vi "DC Supply Control.vi"(8 "error in":errorcluster, 10 "VISA res in":refnum<visa-resource-name>, 11 "HTS Results in":refnum<class "HTS Results.lvclass">) -> (0 "error out":errorcluster, 1 "Supp I":dbl, 2 "VISA res out":refnum<visa-resource-name>, 3 "HTS Results out":refnum<class "HTS Results.lvclass">)   [LabVIEW 2019, in "Results.lvlib" / "HTS Results.lvclass"]
uses:
  HTS Results.lvclass
  HTS Results.lvclass/HTS Results.ctl
  <instrlib>/Agilent 66XX Series/Agilent 66XX Series.lvlib
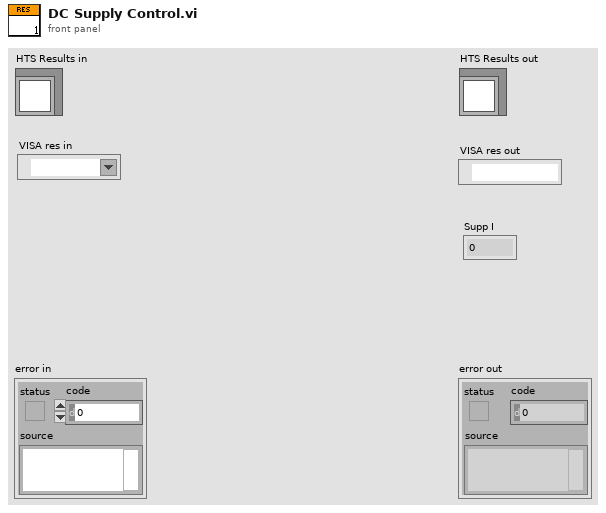
[diagram p1: front panel]
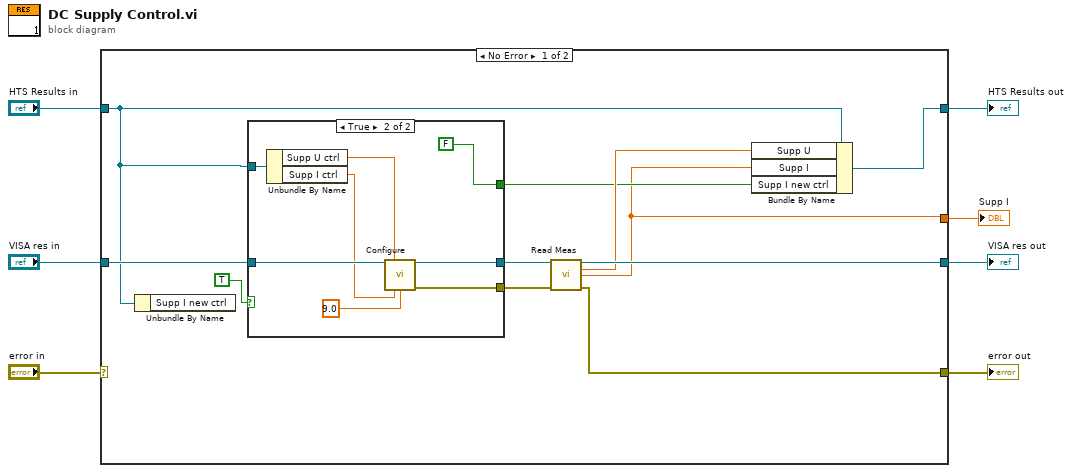
[diagram p0: block diagram]
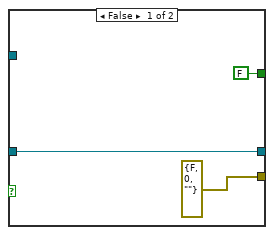
[diagram p2: hidden frame]
diagram:
  n1 = case shown="No Error" "error in" {
    selector: "error in" -> [_ w32]
    tunnel: [w14 w32] -> w6
    tunnel: [w18 w31] -> w4
    tunnel: "HTS Results in" -> [w16 w31]
    tunnel: "VISA res in" -> [w17 w30]
    tunnel: [w15 w30] -> w2
    tunnel: [w8 _] -> w1
    frame No Error {
      n2 = Unbundle By Name(w16) -> ()  [unwired: 1 out]
      n3 = case shown="True" TRUE {
        tunnel: w17 -> [w21 w29]
        tunnel: w16 -> [_ w28]
        tunnel: [w21 w24] -> w13
        tunnel: [errorcluster {"status"=FALSE, "code"=0, "source"=""} ("error out") w23] -> w12
        tunnel: [FALSE ("Supp I new ctrl") FALSE ("Supp I new ctrl")] -> w10
        frame False {
        }
        frame True {
          n4 = Unbundle By Name(w28) -> ("Supp U ctrl"=w27:dbl, "Supp I ctrl"=w26:dbl)
          n5 = call <instrlib>:"Configure.vi"("VISA resource name"=w29, "Voltage(0 Volts)"=w27, "Current(0 Amps)"=w26, "Overvoltage prot value(50 Volts)"=9.0) -> ("VISA resource name out"=w24:refnum<visa-resource-name>, "error out"=w23:errorcluster)  [unwired: 10 in]
        }
      }
      n6 = call <instrlib>:"Read Meas.vi"("VISA resource name"=w13, "error in (no error)"=w12) -> ("VISA resource name out"=w15:refnum<visa-resource-name>, "Voltage (Volts)"=w11:dbl, "Current (Amps)"=w8:dbl, "error out"=w14:errorcluster)  [unwired: 10 in]
      n7 = Bundle By Name(cluster=w16, "Supp U"=w11, "Supp I"=w8, "Supp I new ctrl"=w10) -> (w18:refnum<class "HTS Results.lvclass">)
    }
    frame Error {
    }
  }
  "error out" <- w6
  "HTS Results out" <- w4
  "VISA res out" <- w2
  "Supp I" <- w1
